vi "4-bit DIO .vi"(0 "DIO Refnum 1":refnum<k21>, 1 "DIO Refnum 2":refnum<k21>, 2 "DIO Refnum 3":refnum<k21>, 3 "DIO Refnum 4":refnum<k21>, 5 "DIO OUT[3:0]":u8, 7 "DIO DIR[3:0]":u8) -> (17 "DIO IN[3:0]":u8)   [LabVIEW 2019]
panel:
  # "This VI reads a Boolean value from or writes the value to the specified FPGA I/O item according to the direction of the data flow (DIR).\n- DIR: TRUE - Write data to OUT\n- DIR: FALSE - Read data from IN"
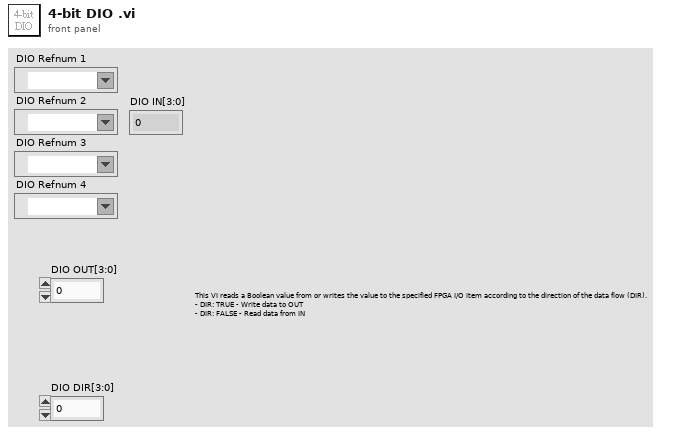
[diagram p1: front panel]
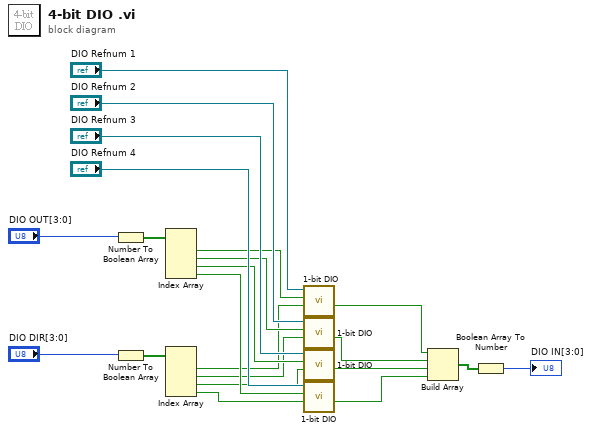
[diagram p0: block diagram]
diagram:
  n1 = Number To Boolean Array(number="DIO OUT[3:0]") -> (Boolean array=w18:bool[])
  n2 = Number To Boolean Array(number="DIO DIR[3:0]") -> (Boolean array=w11:bool[])
  n3 = Index Array(array=w18) -> (element #1=w17:bool, element #2=w16:bool, element #3=w15:bool, element #4=w14:bool)  [unwired: 4 in]
  n4 = Index Array(array=w11) -> (element #1=w10:bool, element #2=w9:bool, element #3=w8:bool, element #4=w7:bool)  [unwired: 4 in]
  n5 = call "1-bit DIO.vi"("DIR"=w10, "OUT"=w17, "DIO Refnum"="DIO Refnum 1") -> ("IN"=w6:bool)  [unwired: 8 in]
  n6 = call "1-bit DIO.vi"("DIR"=w9, "OUT"=w16, "DIO Refnum"="DIO Refnum 2") -> ("IN"=w5:bool)  [unwired: 8 in]
  n7 = call "1-bit DIO.vi"("DIR"=w8, "OUT"=w15, "DIO Refnum"="DIO Refnum 3") -> ("IN"=w3:bool)  [unwired: 8 in]
  n8 = call "1-bit DIO.vi"("DIR"=w7, "OUT"=w14, "DIO Refnum"="DIO Refnum 4") -> ("IN"=w4:bool)  [unwired: 8 in]
  n9 = Build Array(w6, w5, w3, w4) -> (w2:bool[])
  n10 = Boolean Array To Number(Boolean array=w2) -> (number=→"DIO IN[3:0]":u8)
